vi "Sensor_Values.vi"() -> ()   [LabVIEW 2019]
panel:
  out "Zero Pose Estimation":bool
  in  "Camera_Ball_Area":dbl
  in  "Camera_Ball_X":dbl
  out "Camera_Ball_Detected":bool
  in  "Robot_X(ft)":dbl
  in  "Robot_Y(ft)":dbl
  out "IR_10-oclock":bool
  in  "Intake_Velocity(RPM)":dbl
  in  "Spindexer_Velocity(RPM)":dbl
  in  "Spindexer_Position(Rotations)":dbl
  in  "Cowl_Velocity(Degrees/min)":dbl
  in  "Cowl_Position(Degrees)":dbl
  in  "Turret_Relative_Position(Degrees)":dbl
  out "IR_3-oclock":bool
  out "Unjammed":bool
  in  "Turret_Absolute_Position(Native Units)":dbl
  in  "Drive_IMU(Degrees)":dbl
  in  "Climb_IMU":dbl
  in  "Magazine_Position":dbl
  in  "Elevator_Right_Position(Native)":dbl
  in  "Elevator_Left_Position(Native)":dbl
  in  "Climb_Pivot_Position":dbl
  out "Climb_Bottom_Limit":bool
  out "Climb_Top_Limit":bool
  in  "Camera_Area":dbl
  in  "Camera_X_Offset":dbl
  out "Zero_Turret_Spin":bool
  out "IR_8-oclock":bool
  out "IR_5-oclock":bool
  out "IR_12-oclock":bool
  in  "Control_Panel_Velocity(RPM)":dbl
  in  "Control_Panel_Position":dbl
  in  "Turret_Velocity(Degrees/min)":dbl
  in  "Turret_Relative_Position(Native Units)":dbl
  in  "Magazine_Velocity(RPM)":dbl
  in  "Flywheel_Velocity(RPM)":dbl
  in  "Right_Drive_Position(Rotations)":dbl
  in  "Left_Drive_Position(Rotations)":dbl
  in  "Right_Drive_Velocity(RPM)":dbl
  in  "Left_Drive_Velocity(RPM)":dbl
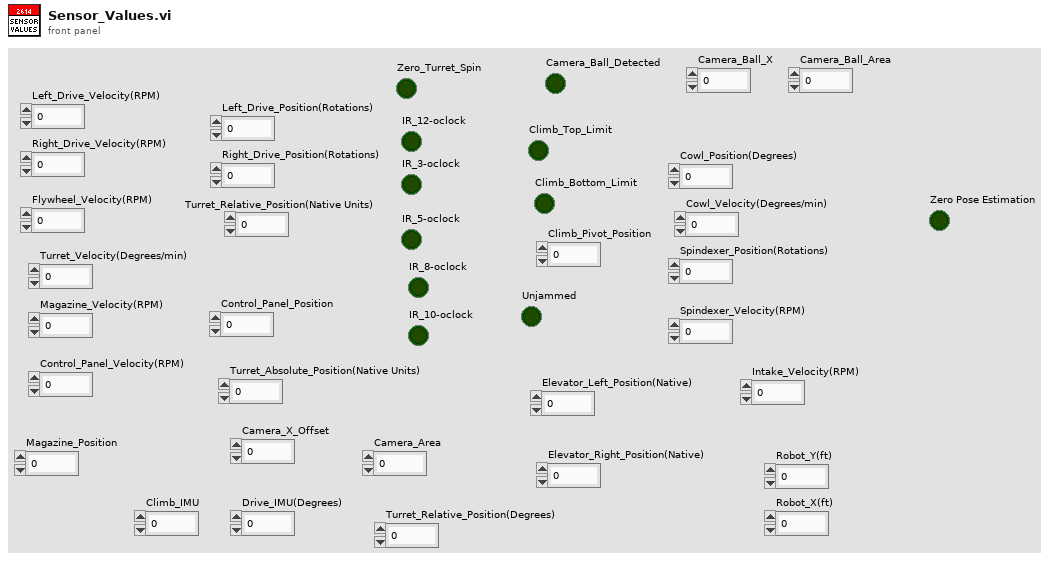
[diagram p1: front panel]
diagram:
